vi "Chrg_dis.vi"(0 "Relay Task":refnum<k21>, 1 "task error in":errorcluster, 2 "Parallel Task in":refnum<k21>, 3 "P task error in":errorcluster, 4 "NHR VISA":refnum<visa-resource-name>, 5 "NHR error in":errorcluster caption="error in (no error)", 6 "Batteryname":string, 7 "Starting Cycle":i32, 8 "Battery Select":i32, 9 "In for loop?":bool, 10 "Capacity (Ah)":dbl format="%#.6g", 11 "For loop i":i32, 12 "C rate Setpoint":dbl format="%#.6g", 13 "Wait time (s)":dbl) -> ()   [LabVIEW 2020]
uses:
  <instrlib>/NH Research Regenerative Test Series/NH Research Regenerative Test Series.lvlib
panel:
  out "Relay error out":errorcluster
  out "Task error out":errorcluster
  out "String":string
  out "Wait2 Elapsed Time (s)":dbl caption="Elapsed Time (s)"
  out "Wait1 Elapsed Time (s)":dbl caption="Elapsed Time (s)"
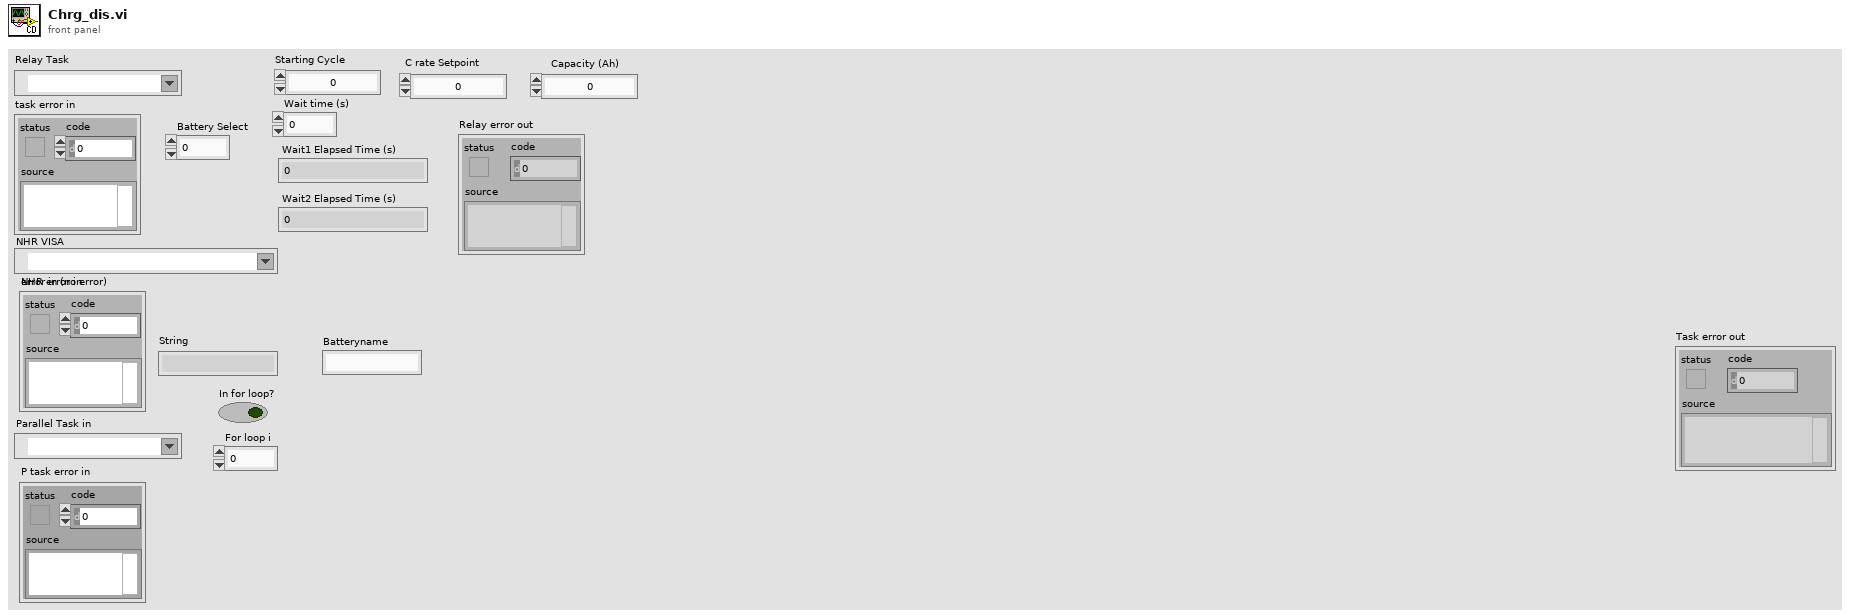
[diagram p1: front panel]
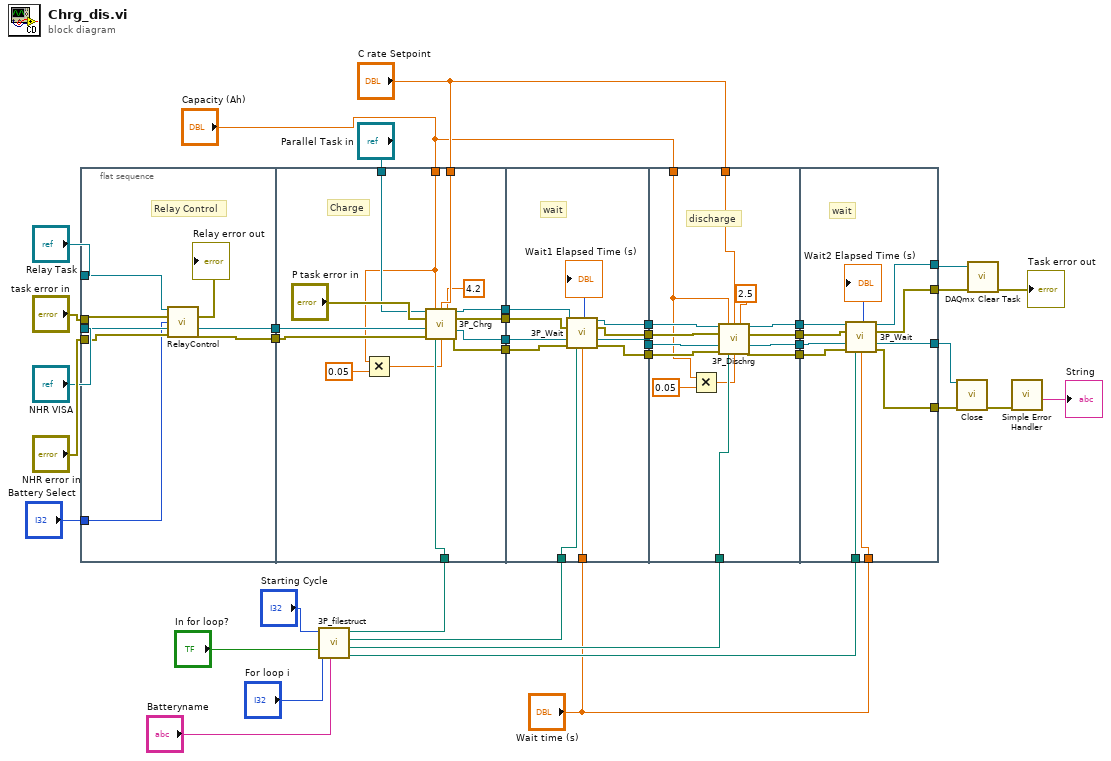
[diagram p0: block diagram]
diagram:
  n1 = flat-sequence {
    tunnel: "NHR error in" -> [w43]
    tunnel: "NHR VISA" -> [w44]
    tunnel: "task error in" -> [w45]
    tunnel: "Relay Task" -> [w46]
    tunnel: [w41] -> w7
    tunnel: [w40] -> w6
    tunnel: "Battery Select" -> [w39]
    tunnel: w37 -> [w52]
    tunnel: "C rate Setpoint" -> [w60]
    tunnel: "Parallel Task in" -> [w57]
    tunnel: [w56] -> w11
    tunnel: [w55] -> w10
    tunnel: [w54] -> w9
    tunnel: [w53] -> w8
    tunnel: w7 -> [w51]
    tunnel: w6 -> [w50]
    tunnel: "Capacity (Ah)" -> [w48]
    tunnel: "Wait time (s)" -> [w71]
    tunnel: [w69] -> w31
    tunnel: [w68] -> w30
    tunnel: [w67] -> w29
    tunnel: [w66] -> w28
    tunnel: w25 -> [w65]
    tunnel: w11 -> [w64]
    tunnel: w10 -> [w63]
    tunnel: w9 -> [w62]
    tunnel: w8 -> [w61]
    tunnel: w31 -> [w85]
    tunnel: w30 -> [w84]
    tunnel: w29 -> [w83]
    tunnel: w28 -> [w82]
    tunnel: "C rate Setpoint" -> [w81]
    tunnel: w26 -> [w80]
    tunnel: [w78] -> w24
    tunnel: [w77] -> w23
    tunnel: [w76] -> w22
    tunnel: [w75] -> w21
    tunnel: "Capacity (Ah)" -> [w72]
    tunnel: w24 -> [w95]
    tunnel: w23 -> [w94]
    tunnel: w22 -> [w93]
    tunnel: w21 -> [w92]
    tunnel: w20 -> [w91]
    tunnel: "Wait time (s)" -> [w90]
    tunnel: [w89] -> w15
    tunnel: [w88] -> w14
    tunnel: [w87] -> w13
    tunnel: [w86] -> w12
    frame #0 {
      # "Relay Control"
      n2 = call "RelayControl.vi"("Relay Task"=w46, "error in"=w45, "Battery Select (0: Off)"=w39, "NHR VISA"=w44, "NHR error in"=w43) -> ("error out"=→"Relay error out":errorcluster, "NHR Visa out"=w41:refnum<visa-resource-name>, "NHR error out"=w40:errorcluster)  [unwired: 8 in]
    }
    frame #1 {
      # "Charge"
      n3 = Multiply(x=w48, y=0.05) -> (x*y=w47:dbl)
      n4 = call "3P_Chrg.vi"("Parallel Task in"=w57, "Capacity (Ah)"=w48, "C rate Setpoint"=w60, "Charge Voltage Setpoint"=4.2, "P task error in"="P task error in", "NHR VISA in"=w51, "NHR error in"=w50, "ChargeCyclePath"=w52, "Current Cutoff"=w47) -> ("parallel task out"=w53:refnum<k21>, "parallel task error out"=w54:errorcluster, "VISA resource name out"=w56:refnum<visa-resource-name>, "NHR error out"=w55:errorcluster)  [unwired: 3 in]
    }
    frame #2 {
      # "wait"
      n5 = call "3P_Wait.vi"("Parallel Task in"=w61, "P task error in"=w62, "NHR VISA in"=w64, "NHR error in"=w63, "Wait Filepath"=w65, "Wait time"=w71) -> ("WaitElapsed Time (s)"=→"Wait1 Elapsed Time (s)":i32, "parallel task out"=w69:refnum<k21>, "parallel task error out"=w68:errorcluster, "NHR Visa Out"=w67:refnum<visa-resource-name>, "NHR error out"=w66:errorcluster)  [unwired: 5 in]
    }
    frame #3 {
      # "discharge"
      n6 = Multiply(x=w72, y=0.05) -> (x*y=w73:dbl)
      n7 = call "3P_Dischrg.vi"("Parallel Task in"=w85, "Capacity (Ah)"=w72, "C rate Setpoint"=w81, "Discharge Voltage Setpoint"=2.5, "P task error in"=w84, "NHR VISA in"=w83, "NHR error in"=w82, "DischargeCyclePath"=w80, "Current Cutoff"=w73) -> ("parallel task out"=w78:refnum<k21>, "parallel task error out"=w77:errorcluster, "VISA resource name out"=w76:refnum<visa-resource-name>, "NHR error out"=w75:errorcluster)  [unwired: 3 in]
    }
    frame #4 {
      # "wait"
      n8 = call "3P_Wait.vi"("Parallel Task in"=w95, "P task error in"=w94, "NHR VISA in"=w93, "NHR error in"=w92, "Wait Filepath"=w91, "Wait time"=w90) -> ("WaitElapsed Time (s)"=→"Wait2 Elapsed Time (s)":i32, "parallel task out"=w89:refnum<k21>, "parallel task error out"=w88:errorcluster, "NHR Visa Out"=w86:refnum<visa-resource-name>, "NHR error out"=w87:errorcluster)  [unwired: 5 in]
    }
  }
  n9 = call "3P_filestruct.vi"("Batteryname"="Batteryname", "For loop i"="For loop i", "In for loop"="In for loop?", "Starting Cycle"="Starting Cycle") -> ("DischargeWaitPath"=w20:path, "DischargeCyclePath"=w26:path, "ChargeWaitPath"=w25:path, "ChargeCyclePath"=w37:path)  [unwired: 3 in, 1 out]
  n10 = call <instrlib>:"Close.vi"("VISA resource name"=w12, "error in (no error)"=w13) -> ("error out"=w16:errorcluster)  [unwired: 13 in]
  n11 = call <vilib>:"DAQmx Clear Task.vi"("task in"=w15, "error in"=w14) -> ("error out"=→"Task error out":errorcluster)  [unwired: 13 in]
  n12 = call <vilib>:"Simple Error Handler.vi"("error in (no error)"=w16) -> ("source out"=→"String":string)  [unwired: 4 in, 4 out]
